vi "VESA 참조경로.vi"(8 "error in (no error)":errorcluster caption="에러 입력(에러 없음)", 11 "이름 또는 상대 경로":string) -> (0 "error out":errorcluster caption="에러 출력", 2 "file or folder exists?":bool caption="파일 또는 폴더가 존재합니까?", 3 "추가된 경로":path)   [LabVIEW 2014]
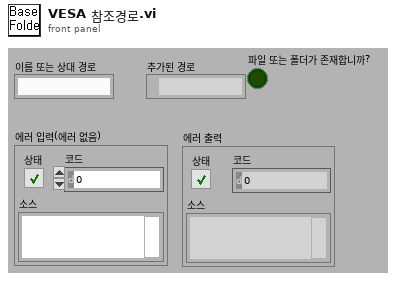
[diagram p1: front panel]
types:
  T1 = enum32{"invalid app kind", "Development System", "Run Time System", "Student Edition", "Embedded LabVIEW", "Evaluation", "Custom"}
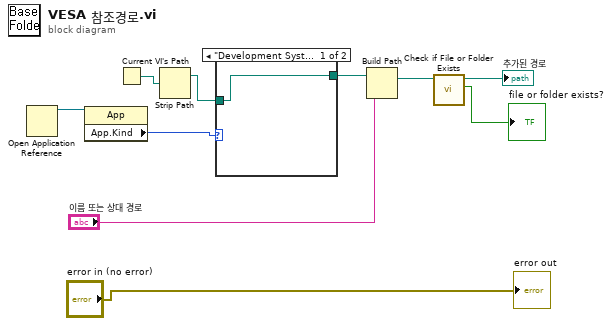
[diagram p0: block diagram]
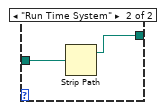
[diagram p2: hidden frame]
diagram:
  n1 = Open Application Reference() -> (3:w8:refnum<vi>)  [unwired: 4 in, 1 out]
  n2 = property class="App"(reference=w8) -> ("App.Kind"=w7:T1)  [unwired: 1 in, 2 out]
  n3 = Current VI's Path() -> (path=w10:path)
  n4 = Strip Path(path=w10) -> (stripped path=w6:path)  [unwired: 1 out]
  n5 = case shown="\"Development System\", 기본" w7 {
    tunnel: w6 -> [w11 w13]
    tunnel: [w11 w12] -> w5
    frame "Development System", Default {
    }
    frame "Run Time System" {
      n6 = Strip Path(path=w13) -> (stripped path=w12:path)  [unwired: 1 out]
    }
  }
  n7 = Build Path(base path=w5, name or relative path="이름 또는 상대 경로") -> (appended path=w4:path)
  n8 = call <vilib>:"Check if File or Folder Exists.vi"("path"=w4) -> ("file or folder exists?"=→"file or folder exists?":bool, "dup path"=→"추가된 경로":path)  [unwired: 8 in, 1 out]
  "error out" <- "error in (no error)"
